vi "Set Custom Error.vi"(7 "append msg to existing error in":bool, 8 "error in":errorcluster, 9 "message in":string, 10 "source in":string, 11 "code in":i32) -> (0 "error out":errorcluster)   [LabVIEW 2022 SP3]
uses:
  <vilib>/regexp/Match Regular Expression.xnode
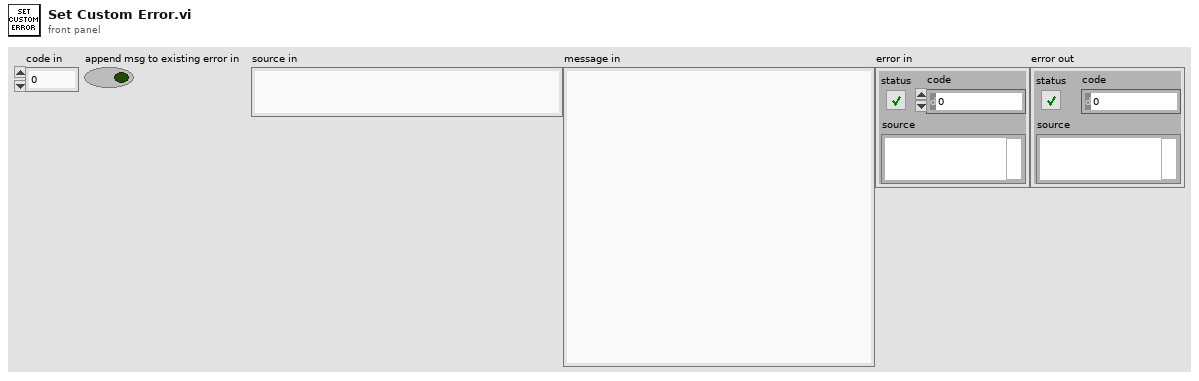
[diagram p1: front panel]
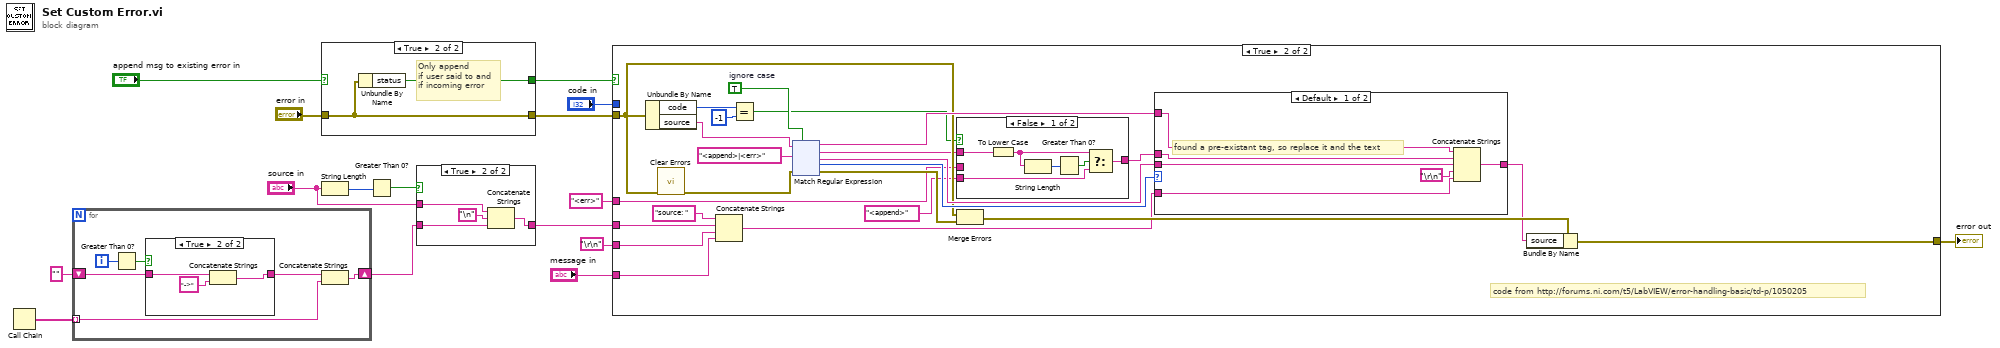
[diagram p0: block diagram]
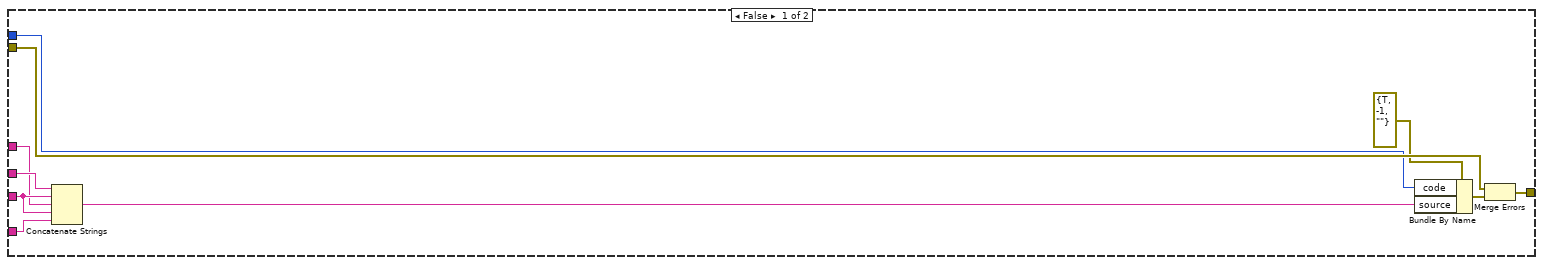
[diagram p5: hidden frame]
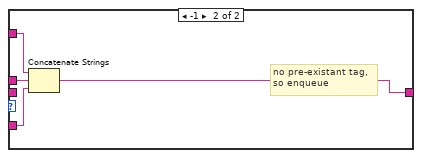
[diagram p7: hidden frame]
diagram:
  n1 = Call Chain() -> (call chain=w7:string[])
  n2 = for {
    tunnel: w7 -> [w17] mode=indexing
    shift-right: [w18] -> w2
    shift-left: "" -> [w22]
    i -> [w21]
    n3 = Greater Than 0?(x=w21) -> (x > 0?=w20:bool)
    n4 = case shown="True" w20 {
      tunnel: [w23 w26] -> w19
      tunnel: w22 -> [w23 w25]
      frame False {
      }
      frame True {
        n5 = Concatenate Strings(w25, "->" ("string")) -> (w26:string)
      }
    }
    n6 = Concatenate Strings(w19, w17) -> (w18:string)
  }
  n7 = case shown="True" "append msg to existing error in" {
    selector: "append msg to existing error in" -> [w27 _]
    tunnel: "error in" -> [w28 w30]
    tunnel: [w27 w29] -> w11
    tunnel: [w28 w30] -> w13
    frame False {
      # "Don't append"
    }
    frame True {
      # "Only append\nif user said to and\nif incoming error"
      n8 = Unbundle By Name(w30) -> ("status"=w29:bool)
    }
  }
  n9 = String Length(string="source in") -> (length=w5:i32)
  n10 = Greater Than 0?(x=w5) -> (x > 0?=w4:bool)
  n11 = case shown="True" w4 {
    tunnel: "source in" -> [_ w34]
    tunnel: w2 -> [w31 w33]
    tunnel: [w31 w32] -> w1
    frame False {
    }
    frame True {
      n12 = Concatenate Strings(w34, "\n", w33) -> (w32:string)
    }
  }
  n13 = case shown="True" w11 {
    tunnel: [w44 w69] -> w16
    tunnel: w13 -> [w43 w56]
    tunnel: "code in" -> [w42 _]
    tunnel: w1 -> [w39 w68]
    tunnel: "message in" -> [w38 w61]
    tunnel: "\r\n" -> [w37 w53]
    tunnel: "<err>" -> [w36 w49]
    frame False {
      n14 = Concatenate Strings(w39, w37, w36, w37, w38) -> (w40:string)
      n15 = Bundle By Name(cluster=errorcluster {"status"=TRUE, "code"=-1, "source"=""} ("error in"), "code"=w42, "source"=w40) -> (w45:errorcluster)
      n16 = Merge Errors(w43, w45) -> (w44:errorcluster)
    }
    frame True {
      w65 = TRUE  # ignore case
      # "code from http://forums.ni.com/t5/LabVIEW/error-handling-basic/td-p/1050205"
      n17 = Unbundle By Name(w56) -> ("code"=w51:i32, "source"=w60:string)
      n18 = call <vilib>:"Clear Errors.vi"("error in (no error)"=w56) -> ("error out"=w59:errorcluster)  [unwired: 5 in, 1 out]
      n19 = Concatenate Strings("source: " ("string"), w68, w53, w61) -> (w55:string)
      n20 = Equal?(x=w51, y=-1) -> (x = y?=w48:bool)
      n21 = xnode "Match Regular Expression"("input string"=w60, "regular expression"="<append>|<err>", "error in"=w59, "ignore case? (F)"=w65) -> ("before match"=w62:string, "whole match"=w50:string, "after match"=w63:string, "offset past match"=w64:i32, "error out"=w58:errorcluster)  [unwired: 2 in]
      n22 = case shown="False" w48 {
        tunnel: w50 -> [w75 _]
        tunnel: [w72 w76] -> w47
        tunnel: w49 -> [_ w76]
        tunnel: "<append>" -> [w70 _]
        frame False {
          n23 = To Lower Case(string=w75) -> (all lower case string=w71:string)
          n24 = String Length(string=w71) -> (length=w74:i32)
          n25 = Greater Than 0?(x=w74) -> (x > 0?=w73:bool)
          n26 = Select(t=w71, s=w73, f=w70) -> (s? t:f=w72:string)
        }
        frame True {
        }
      }
      n27 = Merge Errors(w56, w58) -> (w57:errorcluster)
      n28 = case shown="Default" w64 {
        tunnel: w55 -> [w197 w203]
        tunnel: w63 -> [w198 _]
        tunnel: w62 -> [w199 w202]
        tunnel: [w196 w201] -> w54
        tunnel: w47 -> [w194 w200]
        frame Default {
          # "found a pre-existant tag, so replace it and the text"
          n29 = Concatenate Strings(w199, w194, w198, "\r\n", w197) -> (w196:string)
        }
        frame -1 {
          # "no pre-existant tag,\nso enqueue"
          n30 = Concatenate Strings(w202, w200, w203) -> (w201:string)
        }
      }
      n31 = Bundle By Name(cluster=w57, "source"=w54) -> (w69:errorcluster)
    }
  }
  "error out" <- w16
